vi "Chroma 1905x Series Configure Scanner Channels.vi"(0 "VISA session copy":refnum<visa-resource-name>, 1 "Scanner":T1, 2 "Step":dbl=1.0 min=1.0 max=99.0 step=1.0, 3 "error in":T2, 4 "Mode":u16(ring) items=["AC", "DC", "IR"]) -> (5 "VISA session":refnum<visa-resource-name>, 6 "error out":T2)   [LabVIEW 2025]
uses:
  <instrlib>/Chroma 19052/Chroma 19052.lvlib
panel:
  in  "Box Number":dbl=1.0 min=1.0 max=8.0 step=1.0
  # "Configure Scanner Channels"
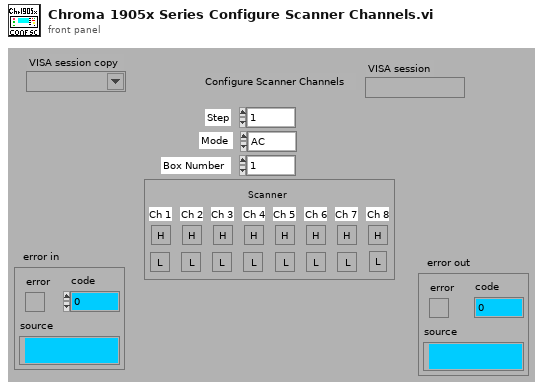
[diagram p1: front panel]
types:
  T1 = cluster{"Ch 3":bool, "Ch 1":bool, "Ch 3 copy":bool, "Ch 2":bool, "Ch 3 copy 2":bool, "Ch 3":bool, "Ch 3 copy 4":bool, "Ch 4":bool, "Ch 3 copy 5":bool, "Ch 5":bool, "Ch 3 copy 6":bool, "Ch 6":bool, "Ch 3 copy 7":bool, "Ch 7":bool, "Ch 3 copy 8":bool, "Ch 8":bool}
  T2 = cluster{"error":bool, "code":i8, "source":string}
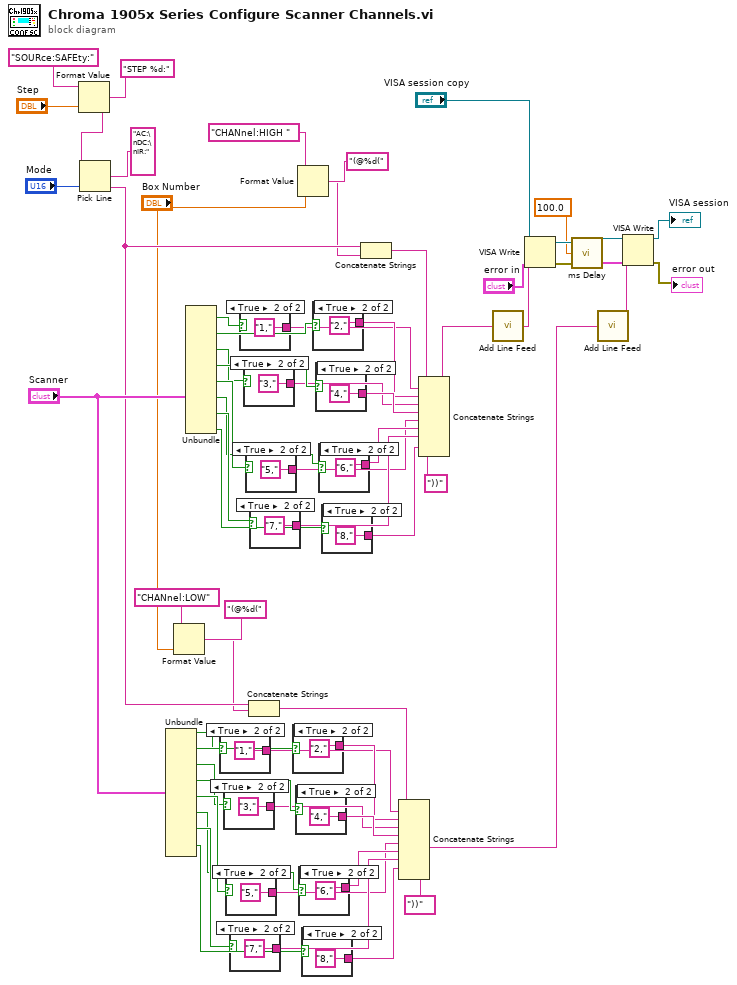
[diagram p0: block diagram]
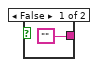
[diagram p2: hidden frame]
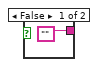
[diagram p3: hidden frame]
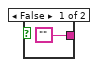
[diagram p4: hidden frame]
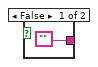
[diagram p5: hidden frame]
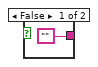
[diagram p6: hidden frame]
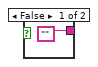
[diagram p7: hidden frame]
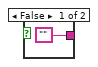
[diagram p8: hidden frame]
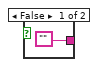
[diagram p9: hidden frame]
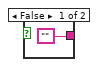
[diagram p10: hidden frame]
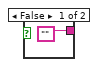
[diagram p11: hidden frame]
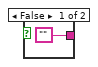
[diagram p12: hidden frame]
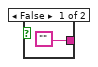
[diagram p13: hidden frame]
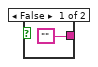
[diagram p14: hidden frame]
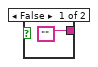
[diagram p15: hidden frame]
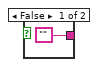
[diagram p16: hidden frame]
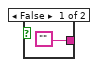
[diagram p17: hidden frame]
diagram:
  n1 = Format Value(string ("")="SOURce:SAFEty:", format string="STEP %d:", value (0)="Step") -> (output string=w58:string)
  n2 = Pick Line(string ("")=w58, multi-line string="AC:\nDC:\nIR:", line index="Mode") -> (output string=w20:string)
  n3 = Unbundle("Scanner") -> ("Ch 3"=w34:bool, "Ch 3 copy"=w35:bool, "Ch 3 copy 2"=w36:bool, "Ch 3 copy 4"=w37:bool, "Ch 3 copy 5"=w38:bool, "Ch 3 copy 6"=w39:bool, "Ch 3 copy 7"=w40:bool, "Ch 3 copy 8"=w41:bool)  [unwired: 8 out]
  n4 = Format Value(string ("")="CHANnel:LOW" ("format string"), format string="(@%d(", value (0)="Box Number") -> (output string=w13:string)
  n5 = Unbundle("Scanner") -> ("Ch 1"=w50:bool, "Ch 2"=w51:bool, "Ch 3"=w52:bool, "Ch 4"=w53:bool, "Ch 5"=w54:bool, "Ch 6"=w55:bool, "Ch 7"=w56:bool, "Ch 8"=w57:bool)  [unwired: 8 out]
  n6 = case shown="True" w34 {
    tunnel: ["" "1,"] -> w26
    frame False {
    }
    frame True {
    }
  }
  n7 = case shown="True" w36 {
    tunnel: ["" "3,"] -> w28
    frame False {
    }
    frame True {
    }
  }
  n8 = case shown="True" w38 {
    tunnel: ["" "5,"] -> w30
    frame False {
    }
    frame True {
    }
  }
  n9 = case shown="True" w40 {
    tunnel: ["" "7,"] -> w32
    frame False {
    }
    frame True {
    }
  }
  n10 = case shown="True" w50 {
    tunnel: ["" "1,"] -> w42
    frame False {
    }
    frame True {
    }
  }
  n11 = case shown="True" w52 {
    tunnel: ["" "3,"] -> w44
    frame False {
    }
    frame True {
    }
  }
  n12 = case shown="True" w54 {
    tunnel: ["" "5,"] -> w46
    frame False {
    }
    frame True {
    }
  }
  n13 = Concatenate Strings(w20, w13) -> (w21:string)
  n14 = case shown="True" w56 {
    tunnel: ["" "7,"] -> w48
    frame False {
    }
    frame True {
    }
  }
  n15 = case shown="True" w35 {
    tunnel: ["" "2,"] -> w27
    frame False {
    }
    frame True {
    }
  }
  n16 = case shown="True" w37 {
    tunnel: ["" "4,"] -> w29
    frame False {
    }
    frame True {
    }
  }
  n17 = Format Value(string ("")="CHANnel:HIGH " ("format string"), format string="(@%d(", value (0)="Box Number") -> (output string=w16:string)
  n18 = case shown="True" w39 {
    tunnel: ["" "6,"] -> w31
    frame False {
    }
    frame True {
    }
  }
  n19 = case shown="True" w41 {
    tunnel: ["" "8,"] -> w33
    frame False {
    }
    frame True {
    }
  }
  n20 = case shown="True" w51 {
    tunnel: ["" "2,"] -> w43
    frame False {
    }
    frame True {
    }
  }
  n21 = case shown="True" w53 {
    tunnel: ["" "4,"] -> w45
    frame False {
    }
    frame True {
    }
  }
  n22 = case shown="True" w55 {
    tunnel: ["" "6,"] -> w47
    frame False {
    }
    frame True {
    }
  }
  n23 = case shown="True" w57 {
    tunnel: ["" "8,"] -> w49
    frame False {
    }
    frame True {
    }
  }
  n24 = Concatenate Strings(w20, w16) -> (w25:string)
  n25 = Concatenate Strings(w21, w26, w27, w28, w29, w30, w31, w32, w33, "))") -> (w1:string)
  n26 = Concatenate Strings(w25, w42, w43, w44, w45, w46, w47, w48, w49, "))") -> (w4:string)
  n27 = call <instrlib>:"Add Line Feed.vi"("Cmdstring"=w4) -> ("Concatenated String"=w3:string)
  n28 = VISA Write(VISA resource name="VISA session copy", write buffer=w3, error in (no error)="error in") -> (VISA resource name out=w9:refnum<visa-resource-name>, error out=w10:errorcluster)  [unwired: 1 out]
  n29 = call <instrlib>:"ms Delay.vi"("error in"=w10, "Time Delay S"=100.0, "inst handle in"=w9) -> ("error out"=w7:T2, "inst handle Out"=w8:refnum<visa-resource-name>)
  n30 = call <instrlib>:"Add Line Feed.vi"("Cmdstring"=w1) -> ("Concatenated String"=w2:string)
  n31 = VISA Write(VISA resource name=w8, write buffer=w2, error in (no error)=w7) -> (VISA resource name out=→"VISA session":refnum<visa-resource-name>, error out=→"error out":errorcluster)  [unwired: 1 out]
